vi "Day 3.2 - Calculate life support rating.vi"(11 "input":string[](array[string])) -> (3 "output":u32)   [LabVIEW 2021]
panel:
  out "CO2 scrub":u32
  out "O2 gen":u32
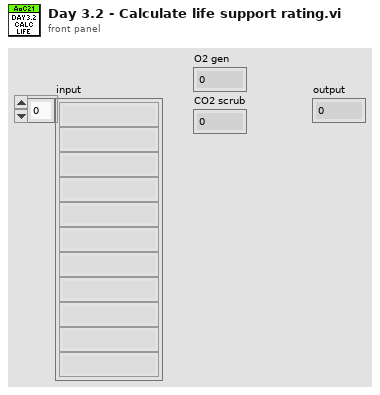
[diagram p1: front panel]
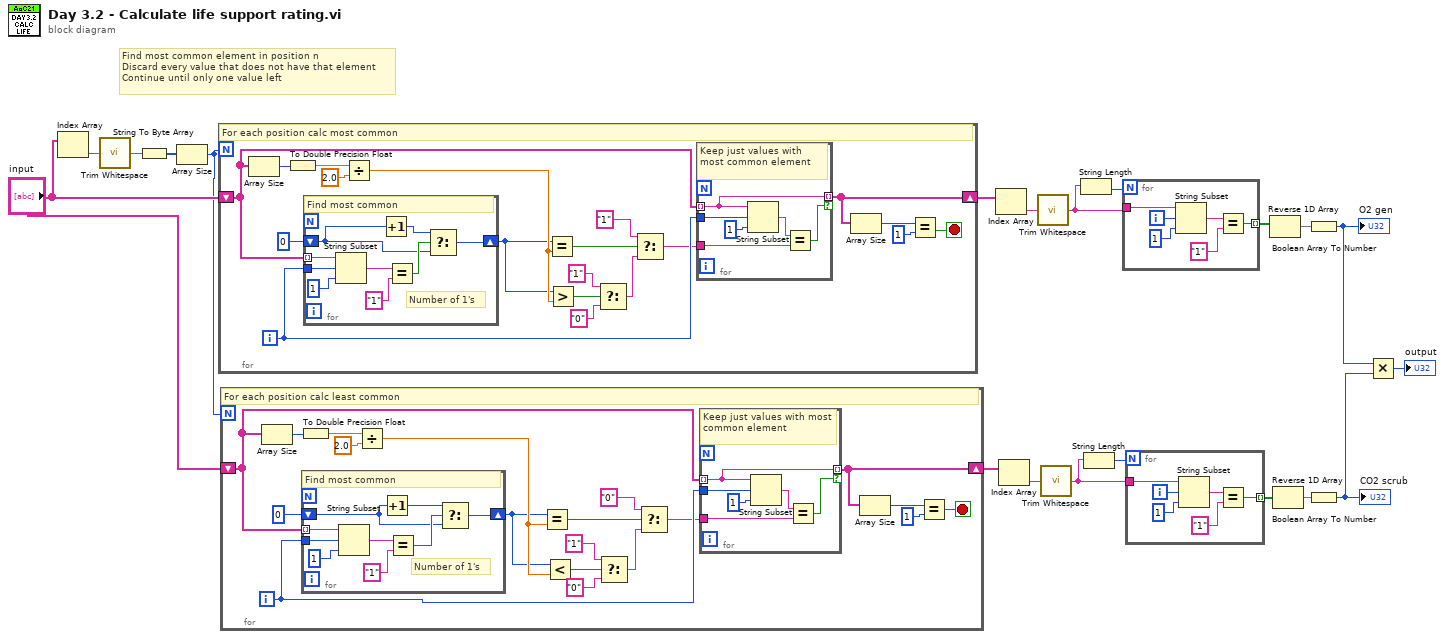
[diagram p0: block diagram]
diagram:
  # "Find most common element in position n\nDiscard every value that does not have that element\nContinue until only one value left"
  n1 = Index Array(array="input") -> (element=w19:string)  [unwired: 1 in]
  n2 = call <vilib>:"Trim Whitespace.vi"("string"=w19) -> ("trimmed string"=w20:string)  [unwired: 1 in]
  n3 = String To Byte Array(string=w20) -> (unsigned byte array=w18:u8[])
  n4 = Array Size(array=w18) -> (size(s)=w14:i32)
  n5 = for {
    N: w14 -> [_]
    shift-right: [w22] -> w4
    shift-left: "input" -> [w24]
    i -> [w32]
    stop <- w34 stop-if-true
    # "For each position calc most common"
    n6 = Array Size(array=w24) -> (size(s)=w23:i32)
    n7 = To Double Precision Float(number=w23) -> (double precision float=w39:dbl)
    n8 = for {
      tunnel: w24 -> [w54] mode=indexing
      tunnel: w32 -> [w53]
      shift-right: [w48] -> w29
      shift-left: 0 -> [w46]
      # "Number of 1's"
      # "Find most common"
      n9 = String Subset(string=w54, offset (0)=w53, length (rest)=1 ("length (rest)")) -> (substring=w51:string)
      n10 = Increment(x=w46) -> (x+1=w47:i32)
      n11 = Equal?(x=w51, y="1") -> (x = y?=w49:bool)
      n12 = Select(t=w47, s=w49, f=w46) -> (s? t:f=w48:i32)
    }
    n13 = Divide(x=w39, y=2.0) -> (x/y=w37:dbl)
    n14 = Equal?(x=w29, y=w37) -> (x = y?=w28:bool)
    n15 = Greater?(x=w29, y=w37) -> (0:w31:bool)
    n16 = Select(t="1" ("y"), s=w31, f="0" ("y")) -> (s? t:f=w26:string)
    n17 = Select(t="1" ("y"), s=w28, f=w26) -> (s? t:f=w25:string)
    n18 = for {
      tunnel: w24 -> [w43] mode=indexing
      tunnel: [w43] -> w22 mode=indexing if=w40
      tunnel: w32 -> [w42]
      tunnel: w25 -> [w41]
      # "Keep just values with most common element"
      n19 = String Subset(string=w43, offset (0)=w42, length (rest)=1 ("length (rest)")) -> (substring=w44:string)
      n20 = Equal?(x=w44, y=w41) -> (x = y?=w40:bool)
    }
    n21 = Array Size(array=w22) -> (size(s)=w36:i32)
    n22 = Equal?(x=w36, y=1) -> (x = y?=w34:bool)
  }
  n23 = for {
    N: w14 -> [_]
    shift-right: [w58] -> w11
    shift-left: "input" -> [w60]
    i -> [w66]
    stop <- w68 stop-if-true
    # "For each position calc least common"
    n24 = Array Size(array=w60) -> (size(s)=w59:i32)
    n25 = To Double Precision Float(number=w59) -> (double precision float=w73:dbl)
    n26 = for {
      tunnel: w60 -> [w88] mode=indexing
      tunnel: w66 -> [w87]
      shift-right: [w82] -> w64
      shift-left: 0 -> [w80]
      # "Number of 1's"
      # "Find most common"
      n27 = String Subset(string=w88, offset (0)=w87, length (rest)=1 ("length (rest)")) -> (substring=w85:string)
      n28 = Increment(x=w80) -> (x+1=w81:i32)
      n29 = Equal?(x=w85, y="1") -> (x = y?=w83:bool)
      n30 = Select(t=w81, s=w83, f=w80) -> (s? t:f=w82:i32)
    }
    n31 = Divide(x=w73, y=2.0) -> (x/y=w71:dbl)
    n32 = Equal?(x=w64, y=w71) -> (x = y?=w63:bool)
    n33 = Less?(x=w64, y=w71) -> (x < y?=w65:bool)
    n34 = Select(t="1" ("y"), s=w65, f="0" ("y")) -> (s? t:f=w62:string)
    n35 = Select(t="0" ("y"), s=w63, f=w62) -> (s? t:f=w61:string)
    n36 = for {
      tunnel: w60 -> [w77] mode=indexing
      tunnel: [w77] -> w58 mode=indexing if=w74
      tunnel: w66 -> [w76]
      tunnel: w61 -> [w75]
      # "Keep just values with most common element"
      n37 = String Subset(string=w77, offset (0)=w76, length (rest)=1 ("length (rest)")) -> (substring=w78:string)
      n38 = Equal?(x=w78, y=w75) -> (x = y?=w74:bool)
    }
    n39 = Array Size(array=w58) -> (size(s)=w70:i32)
    n40 = Equal?(x=w70, y=1) -> (x = y?=w68:bool)
  }
  n41 = Index Array(array=w4) -> (element=w7:string)  [unwired: 1 in]
  n42 = Index Array(array=w11) -> (element=w12:string)  [unwired: 1 in]
  n43 = call <vilib>:"Trim Whitespace.vi"("string"=w7) -> ("trimmed string"=w5:string)  [unwired: 1 in]
  n44 = call <vilib>:"Trim Whitespace.vi"("string"=w12) -> ("trimmed string"=w9:string)  [unwired: 1 in]
  n45 = String Length(string=w5) -> (length=w6:i32)
  n46 = String Length(string=w9) -> (length=w10:i32)
  n47 = for {
    N: w6 -> [_]
    tunnel: [w93] -> w3 mode=indexing
    tunnel: w5 -> [w92]
    i -> [w91]
    n48 = String Subset(string=w92, offset (0)=w91, length (rest)=1 ("length (rest)")) -> (substring=w89:string)
    n49 = Equal?(x=w89, y="1") -> (x = y?=w93:bool)
  }
  n50 = for {
    N: w10 -> [_]
    tunnel: [w99] -> w8 mode=indexing
    tunnel: w9 -> [w98]
    i -> [w97]
    n51 = String Subset(string=w98, offset (0)=w97, length (rest)=1 ("length (rest)")) -> (substring=w95:string)
    n52 = Equal?(x=w95, y="1") -> (x = y?=w99:bool)
  }
  n53 = Reverse 1D Array(array=w3) -> (reversed array=w2:bool[])
  n54 = Reverse 1D Array(array=w8) -> (reversed array=w1:bool[])
  n55 = Boolean Array To Number(Boolean array=w2) -> (number=w16:u32)
  "O2 gen" <- w16
  n56 = Boolean Array To Number(Boolean array=w1) -> (number=w13:u32)
  "CO2 scrub" <- w13
  n57 = Multiply(x=w16, y=w13) -> (x*y=→"output":u32)
